vi "KalmanFilterLatencyComp_AddObserverState.vi"(6 "TimeStamp_Sec":dbl, 8 "Local Y":T2, 9 "U":T2, 10 "Observer":T1, 11 "in KalmanFilterLatencyCompensator":T5) -> (3 "out KalmanFilterLatencyCompensator":T5)   [LabVIEW 2019, in "Trajectory_Library.lvlib"]
doc: "Add past observer states to the observer snapshots list.\n \nInputs: \n - KalmanLatencyComp -- Data cluster\n - observer -- The observer. (Uncented Kalman Filter)\n - u -- The input matrix at the timestamp.\n - localY -- The local output matrix at the timestamp\n - timestampSeconds -- The timesnap of the state.\n\nOutputs:\n - outKalmanLatencyComp -- updated data cluster"
uses:
  Trajectory_Library.lvlib
  KALMAN_FILTER_LATENCY_COMP.ctl
  OBSERVER_SNAP_LIST_ITEM.ctl
  OBSERVER_SNAPSHOT.ctl
  <vilib>/Analysis/Matrix/Datatypes/RealMatrix.ctl
  UNSCENTED_KALMAN_FILTER.ctl
  MERWE_SCALED_SIGMA_PTS.ctl
  CALLBACK_FUNC_TYPE.ctl
  <vilib>/Analysis/Matrix/NI_Matrix.lvlib
panel:
  # "Inputs"
  # "Local Measurements"
  # "State Estimate <Statess,1>"
  # "<States, States>"
  # "<States, ?>"
  # "<Statess,  States>"
  # "<Outputs, Outputs>"
  # "<?, 1>"
  # "<?, 1>"
  # "<Statess,1>"
  # "<States, States>"
  # "<Inputs, 1>"
  # "<Outputs,  1>"
  # "<Statess,1>"
  # "<States, States>"
  # "<Inputs, 1>"
  # "<Outputs,  1>"
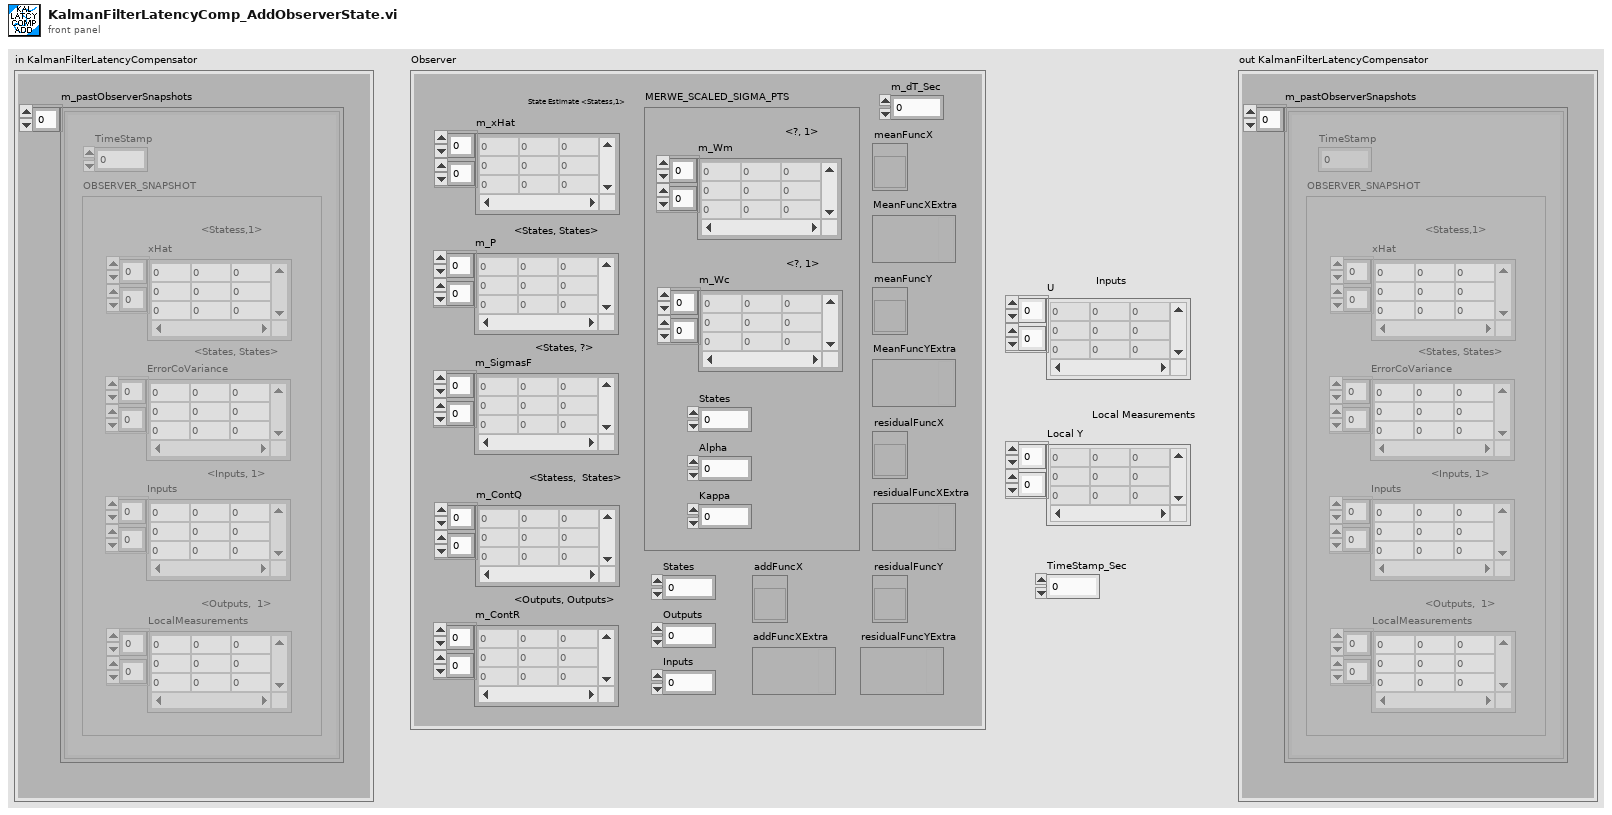
[diagram p1: front panel]
types:
  T1 = typedef "Trajectory_Library.lvlib/UNSCENTED_KALMAN_FILTER.ctl" = cluster{"m_P":T2, "m_xHat":T2, "States":i32, "Outputs":i32, "m_ContR":T2, "m_ContQ":T2, "m_SigmasF":T2, "m_dT_Sec":dbl, "MERWE_SCALED_SIGMA_PTS":T3, "meanFuncX":T4, "meanFuncY":T4, "residualFuncX":T4, "residualFuncY":T4, "addFuncX":T4, "addFuncXExtra":variant, "residualFuncYExtra":variant, "residualFuncXExtra":variant, "MeanFuncYExtra":variant, "MeanFuncXExtra":variant, "Inputs":i32}
  T2 = typedef "NI_Matrix.lvlib/RealMatrix.ctl" = dbl[][]
  T3 = typedef "Trajectory_Library.lvlib/MERWE_SCALED_SIGMA_PTS.ctl" = cluster{"m_Wm":T2, "States":i32, "Alpha":dbl, "m_Wc":T2, "Kappa":i32}
  T4 = typedef "Trajectory_Library.lvlib/CALLBACK_FUNC_TYPE.ctl" = refnum<vi>
  T5 = typedef "Trajectory_Library.lvlib/KALMAN_FILTER_LATENCY_COMP.ctl" = cluster{"m_pastObserverSnapshots ":T6[]}
  T6 = typedef "Trajectory_Library.lvlib/OBSERVER_SNAP_LIST_ITEM.ctl" = cluster{"TimeStamp":dbl, "OBSERVER_SNAPSHOT":T7}
  T7 = typedef "Trajectory_Library.lvlib/OBSERVER_SNAPSHOT.ctl" = cluster{"ErrorCoVariance":T2, "xHat":T2, "LocalMeasurements":T2, "Inputs":T2}
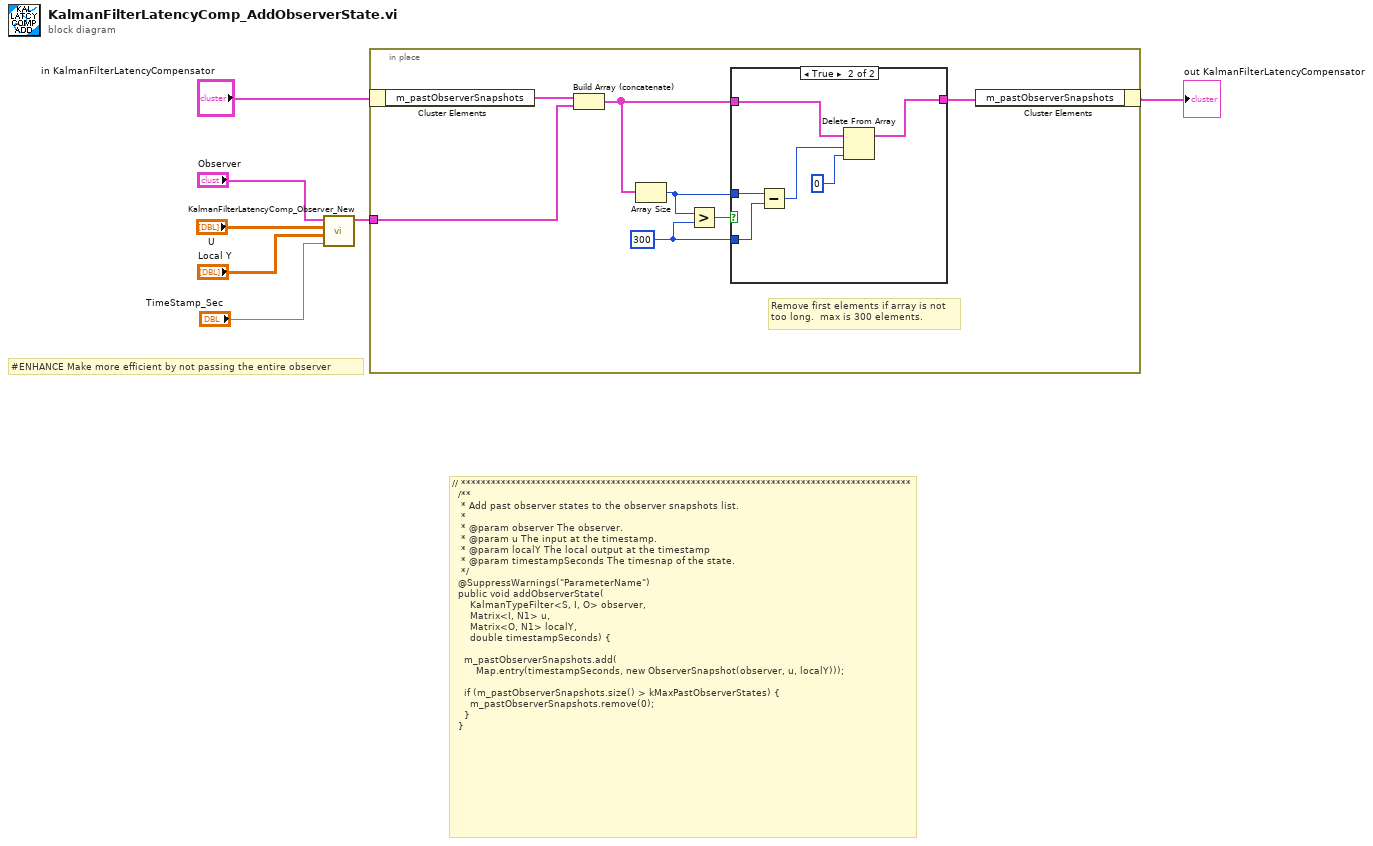
[diagram p0: block diagram]
diagram:
  # "#ENHANCE Make more efficient by not passing the entire observer"
  # "// ******************************************************************************************\n  /**\n   * Add past observer states to the observer snapshots list.\n   *\n   * @param observer The observer.\n   * @param u The input at the timestamp.\n   * @param localY The local output at the timestamp\n   * @param timestampSeconds The timesnap of the state.\n   */\n  @SuppressWarnings(\"ParameterName\")\n  public void addObserverState(\n      KalmanTypeFilter<S, I, O> observer,\n      Matrix<I, N1> u,\n      Matrix<O, N1> localY,\n      double timestampSeconds) {\n\n    m_pastObserverSnapshots.add(\n        Map.entry(timestampSeconds, new ObserverSnapshot(observer, u, localY)));\n\n    if (m_pastObserverSnapshots.size() > kMaxPastObserverStates) {\n      m_pastObserverSnapshots.remove(0);\n    }\n  }"
  n1 = call "KalmanFilterLatencyComp_Observer_New.vi"("TimeStamp_Sec"="TimeStamp_Sec", "LocalY"="Local Y", "U"="U", "Observer"="Observer") -> ("OBSERVER_LIST_ITEM"=w5:T6)  [unwired: 7 in]
  n2 = in-place {
    in-place-border: w5 -> [w13]
    w8 = 300 ("y")
    # "Remove first elements if array is not\ntoo long.  max is 300 elements."
    n3 = in-place-cluster #1("in KalmanFilterLatencyCompensator") -> ("m_pastObserverSnapshots"=w14:T6[])
    n4 = Build Array (concatenate)(w14, w13) -> (w11:T6[])
    n5 = Array Size(array=w11) -> (size(s)=w9:i32)
    n6 = Greater?(x=w9, y=w8) -> (0:w12:bool)
    n7 = case shown="True" w12 {
      tunnel: w11 -> [w15 w17]
      tunnel: [w15 w16] -> w10
      tunnel: w9 -> [_ w21]
      tunnel: w8 -> [_ w20]
      frame False {
      }
      frame True {
        n8 = Subtract(x=w21, y=w20) -> (x-y=w19:i32)
        n9 = Delete From Array(array=w17, length=w19, index=0) -> (array with subset deleted=w16:T6[])  [unwired: 1 out]
      }
    }
    n10 = in-place-cluster #1("m_pastObserverSnapshots"=w10) -> (→"out KalmanFilterLatencyCompensator":T5)
  }
